vi "Reports.Results, Split Desctription to Summary and Details.vi"(10 "Delimiters":string[](array[string])=["|", "\t", "\n"], 11 "Description":string) -> (2 "Details":string, 3 "Summary Description":string)   [LabVIEW 2019]
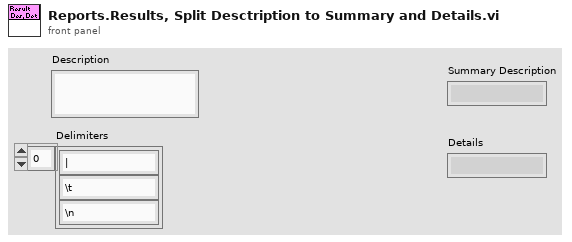
[diagram p1: front panel]
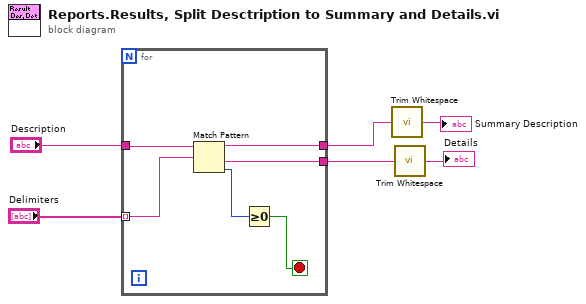
[diagram p0: block diagram]
diagram:
  n1 = for {
    tunnel: "Description" -> [w12]
    tunnel: "Delimiters" -> [w11] mode=indexing
    tunnel: [w10] -> w2
    tunnel: [w9] -> w1
    stop <- w7 stop-if-true
    n2 = Match Pattern(string=w12, regular expression=w11) -> (before substring=w10:string, after substring=w9:string, offset past match=w8:i32)  [unwired: 1 in, 1 out]
    n3 = Greater Or Equal To 0?(x=w8) -> (x >= 0?=w7:bool)
  }
  n4 = call <vilib>:"Trim Whitespace.vi"("string"=w2) -> ("trimmed string"=→"Summary Description":string)  [unwired: 1 in]
  n5 = call <vilib>:"Trim Whitespace.vi"("string"=w1) -> ("trimmed string"=→"Details":string)  [unwired: 1 in]
